vi "SP Calculate Inverse TP Matrices.vi"(10 "T-Parameters":T1) -> (2 "T-Parameters":T1)   [LabVIEW 2011]
uses:
  TypeDefs/SP TP Data.ctl
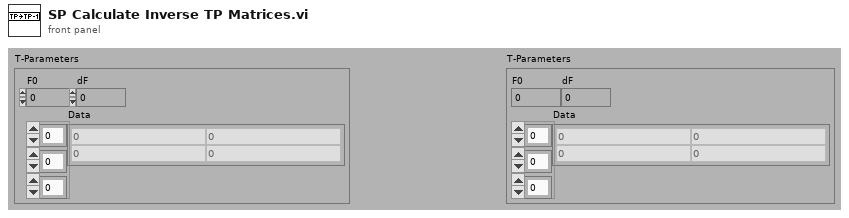
[diagram p1: front panel]
types:
  T1 = typedef "SP TP Data.ctl" = cluster{"F0":dbl, "dF":dbl, "Data":cdb[][][]}
  T2 = typedef "SP Complex Matrix.ctl" = cdb[][]
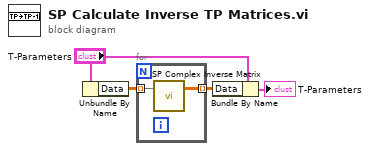
[diagram p0: block diagram]
diagram:
  n1 = Unbundle By Name("T-Parameters") -> ("Data"=w2:cdb[][][])
  n2 = for {
    tunnel: w2 -> [w6] mode=indexing
    tunnel: [w5] -> w4 mode=indexing
    n3 = call "SP Complex Inverse Matrix.vi"("Input Matrix"=w6) -> ("Inverse Matrix"=w5:T2)  [unwired: 2 out]
  }
  n4 = Bundle By Name(cluster="T-Parameters", "Data"=w4) -> (→"T-Parameters":T1)
